vi "Get Object Size.vi"(6 "Version ID":string, 8 "error in (no error)":errorcluster, 9 "Bucket":string, 10 "Path":string) -> (0 "error out":errorcluster, 3 "Object Size (bytes)":u64)   [LabVIEW 2011, in "LV Interface for Amazon S3.lvlib"]
doc: "This operation <B>returns Object size</B> (in bytes). <B>Note:</B> To determine object size, the last byte of the object is retreived via a Get Object request."
uses:
  LV Interface for Amazon S3.lvlib
  Typedefs/AMZ_S3_API_GET Object Request Parameters.ctl
  Typedefs/AMZ_S3_API_GET Request Range.ctl
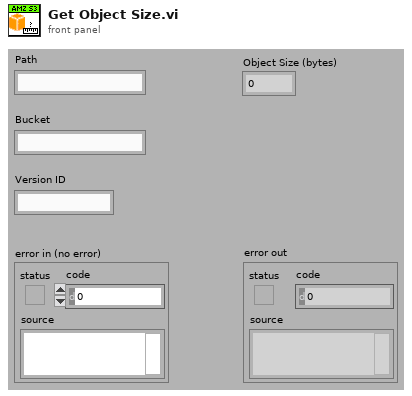
[diagram p1: front panel]
types:
  T1 = typedef "LV Interface for Amazon S3.lvlib/AMZ_S3_API_GET Object Request Parameters.ctl" = cluster{"Range":T2, "If Modified Since":timestamp, "If Unmodified Since":timestamp, "Matching ETag":string, "Nonmatching ETag":string}
  T2 = typedef "LV Interface for Amazon S3.lvlib/AMZ_S3_API_GET Request Range.ctl" = cluster{"Start":i64, "Length":i64}
  T3 = typedef "LV Interface for Amazon S3.lvlib/AMZ_S3_API_GETObjectResult.ctl" = cluster{"Content Length (bytes)":u64, "Content Type":string, "ETag":string, "Delete marker":bool, "Version ID":string, "Object Size (bytes)":u64}
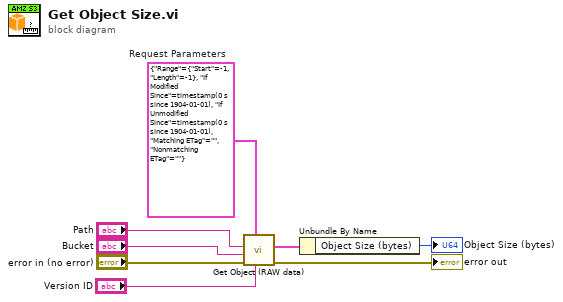
[diagram p0: block diagram]
diagram:
  w8 = T1 {"Range"={"Start"=-1, "Length"=-1}, "If Modified Since"=timestamp(0 s since 1904-01-01), "If Unmodified Since"=timestamp(0 s since 1904-01-01), "Matching ETag"="", "Nonmatching ETag"=""}  # Request Parameters
  n1 = call "Get Object (RAW data).vi"("Version ID"="Version ID", "Request Parameters"=w8, "error in (no error)"="error in (no error)", "Bucket"="Bucket", "Path"="Path") -> ("error out"=→"error out":errorcluster, "GetObjectResult"=w3:T3)  [unwired: 4 in, 1 out]
  n2 = Unbundle By Name(w3) -> ("Object Size (bytes)"=→"Object Size (bytes)":u64)
